vi "ImageAveragingFrames.vi"(6 "new":dbl[](array[numeric]), 8 "Images 2D in":dbl[][](array[numeric]), 9 "Frames grabbed":i32, 10 "y-index":i32, 11 "Frames to Grab":i32) -> (3 "Images 2D out":dbl[][](array[numeric]))   [LabVIEW 2012, in "Image.lvclass"]
uses:
  classes/Image.lvclass
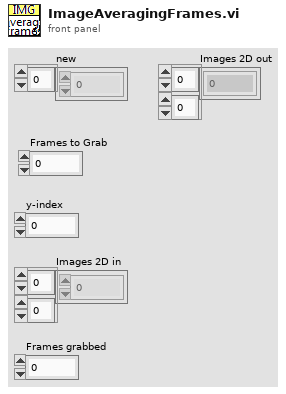
[diagram p1: front panel]
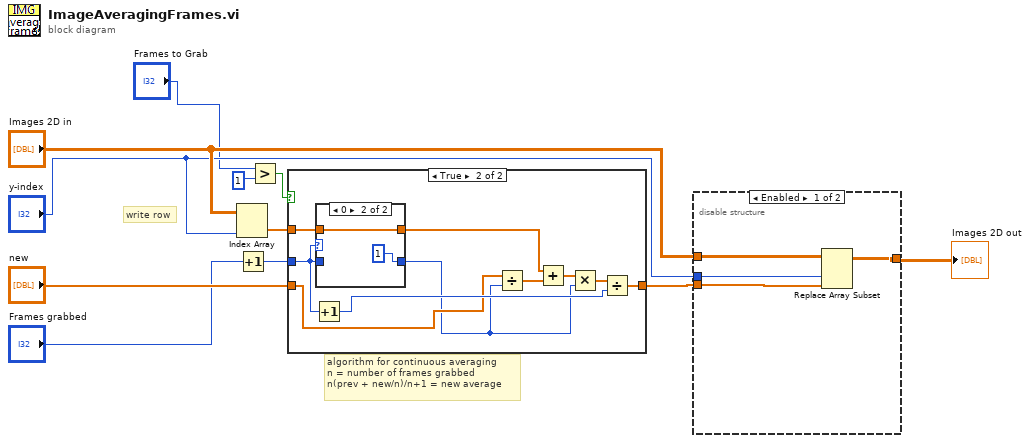
[diagram p0: block diagram]
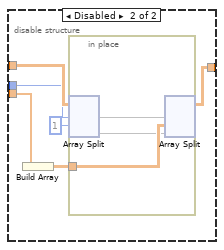
[diagram p2: hidden frame]
diagram:
  # "algorithm for continuous averaging\nn = number of frames grabbed\nn(prev + new/n)/n+1 = new average"
  # "write row"
  n1 = Index Array(array="Images 2D in", index (col)="y-index") -> (element=w8:dbl[])  [unwired: 1 in]
  n2 = Increment(x="Frames grabbed") -> (x+1=w4:i32)
  n3 = Greater?(x="Frames to Grab", y=1) -> (0:w10:bool)
  n4 = case shown="True" w10 {
    tunnel: [w12 w22] -> w7
    tunnel: "new" -> [w12 w20]
    tunnel: w8 -> [_ w14]
    tunnel: w4 -> [_ w13]
    frame False {
    }
    frame True {
      n5 = Increment(x=w13) -> (x+1=w21:i32)
      n6 = case shown="0" w13 {
        tunnel: w13 -> [w24 _]
        tunnel: [w24 1 ("Frames grabbed")] -> w18
        tunnel: [w23 w25] -> w15
        tunnel: w14 -> [w23 w25]
        frame 1, Default {
        }
        frame 0 {
        }
      }
      n7 = Divide(x=w20, y=w18) -> (x/y=w16:dbl[])
      n8 = Add(x=w15, y=w16) -> (x+y=w19:dbl[])
      n9 = Multiply(x=w19, y=w18) -> (x*y=w17:dbl[])
      n10 = Divide(x=w17, y=w21) -> (x/y=w22:dbl[])
    }
  }
  n11 = disable-structure shown="Enabled" {
    disable-tunnel: w7 -> [w30 w33]
    disable-tunnel: [w29 w31] -> w6
    disable-tunnel: "Images 2D in" -> [w28 w36]
    disable-tunnel: "y-index" -> [w27 w34]
    frame Enabled {
      n12 = Replace Array Subset(array=w28, new element=w30, index (col)=w27) -> (w29:dbl[][])  [unwired: 1 in]
    }
    frame Disabled {
      n13 = Build Array(w33) -> (w32:dbl[][])
      n14 = in-place {
        in-place-border: w32 -> [w38]
        n15 = in-place-split #1(w36, w34, 1) -> (w39:dbl[][], w37:dbl[][])  [unwired: 1 out]
        n16 = in-place-split #1(w39, w38, w37) -> (w31:dbl[][])  [unwired: 2 out]
      }
    }
  }
  "Images 2D out" <- w6
